vi "Target Context.vi"(10 "Target Name":string, 11 "Project Path":path) -> (1 "Target":refnum<vi>, 2 "Target Context":refnum<vi>, 3 "Project":refnum<vi>)   [LabVIEW 2020, in "Builder Tools.lvlib"]
uses:
  Builder Tools.lvlib
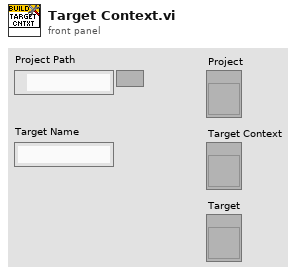
[diagram p1: front panel]
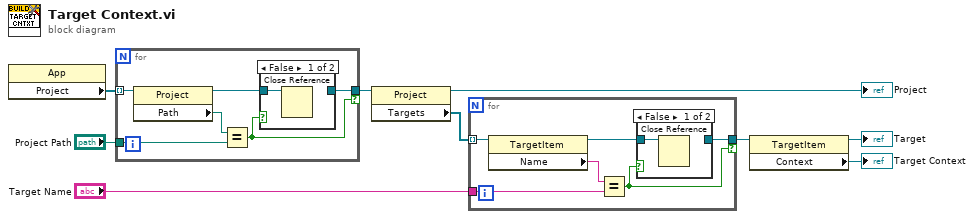
[diagram p0: block diagram]
diagram:
  n1 = property class="App"() -> ("Project"=w9:refnum<vi>[])  [unwired: 2 in, 2 out]
  n2 = for {
    tunnel: w9 -> [w15] mode=indexing
    tunnel: "Project Path" -> [w13]
    tunnel: [w11] -> w7 if=w10
    n3 = property class="Project"(reference=w15) -> (reference out=w12:refnum<vi>, "Path"=w14:path)  [unwired: 1 in, 1 out]
    n4 = Equal?(x=w14, y=w13) -> (x = y?=w10:bool)
    n5 = case shown="False" w10 {
      tunnel: w12 -> [w16 w17]
      tunnel: [_ w17] -> w11
      frame False {
        n6 = Close Reference(reference=w16) -> ()  [unwired: 1 in, 1 out]
      }
      frame True {
      }
    }
  }
  n7 = property class="Project"(reference=w7) -> (reference out=→"Project":refnum<vi>, "Targets"=w6:refnum<vi>[])  [unwired: 1 in, 1 out]
  n8 = for {
    tunnel: w6 -> [w23] mode=indexing
    tunnel: "Target Name" -> [w21]
    tunnel: [w19] -> w3 if=w18
    n9 = property class="TargetItem"(reference=w23) -> (reference out=w20:refnum<vi>, "Name"=w22:string)  [unwired: 1 in, 1 out]
    n10 = Equal?(x=w22, y=w21) -> (x = y?=w18:bool)
    n11 = case shown="False" w18 {
      tunnel: w20 -> [w24 w25]
      tunnel: [_ w25] -> w19
      frame False {
        n12 = Close Reference(reference=w24) -> ()  [unwired: 1 in, 1 out]
      }
      frame True {
      }
    }
  }
  n13 = property class="TargetItem"(reference=w3) -> (reference out=→"Target":refnum<vi>, "Context"=→"Target Context":refnum<vi>)  [unwired: 1 in, 1 out]
